vi "Get Waveform.vi"(0 "VISA resource name":refnum<visa-resource-name>, 1 "First Valid Point":i32, 2 "Last Valid Point":i32, 5 "Source (1: Channel 1)":u16(ring)=1 items=["Channel 1"=1, "Channel 2"=2, "Channel 3"=3, "Channel 4"=4], 7 "Command type (0: byte)":u16(ring) items=["Byte", "Word"], 9 "Number Of Data Points (10000)":i32=10000, 11 "error in (no error)":errorcluster, 12 "Timeout (10000 ms)":u32=10000, 13 "Array (0: DAT1)":u16(ring) items=["DAT1", "DAT2"]) -> (4 "VISA resource name out":refnum<visa-resource-name>, 6 "Waveform Graph":i16[](graph), 15 "error out":errorcluster)   [LabVIEW 2021, in "Siglent SDS 1000 2000 Series.lvlib"]
doc: "Read acquisition waveform from specified source and data block and command format."
uses:
  <instrlib>/Siglent SDS 1000 2000 Series/Siglent SDS 1000 2000 Series.lvlib
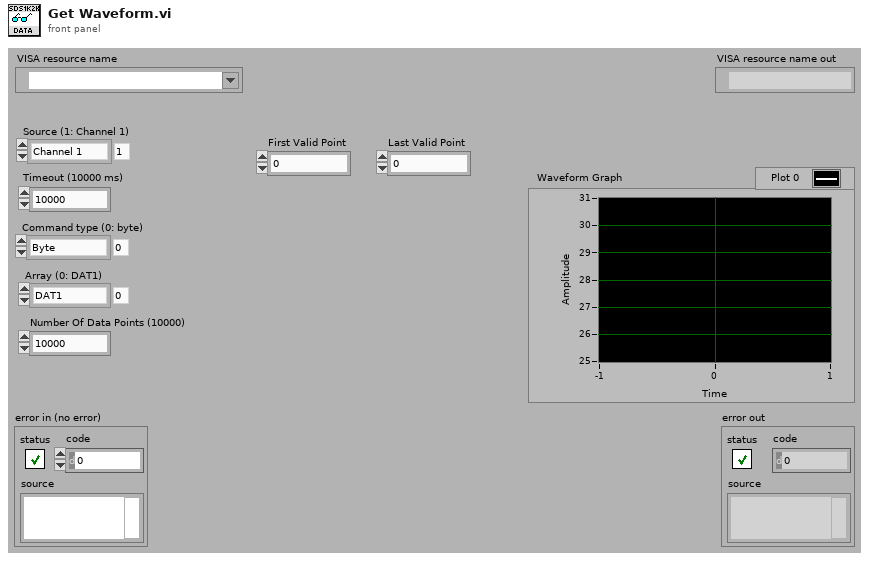
[diagram p1: front panel]
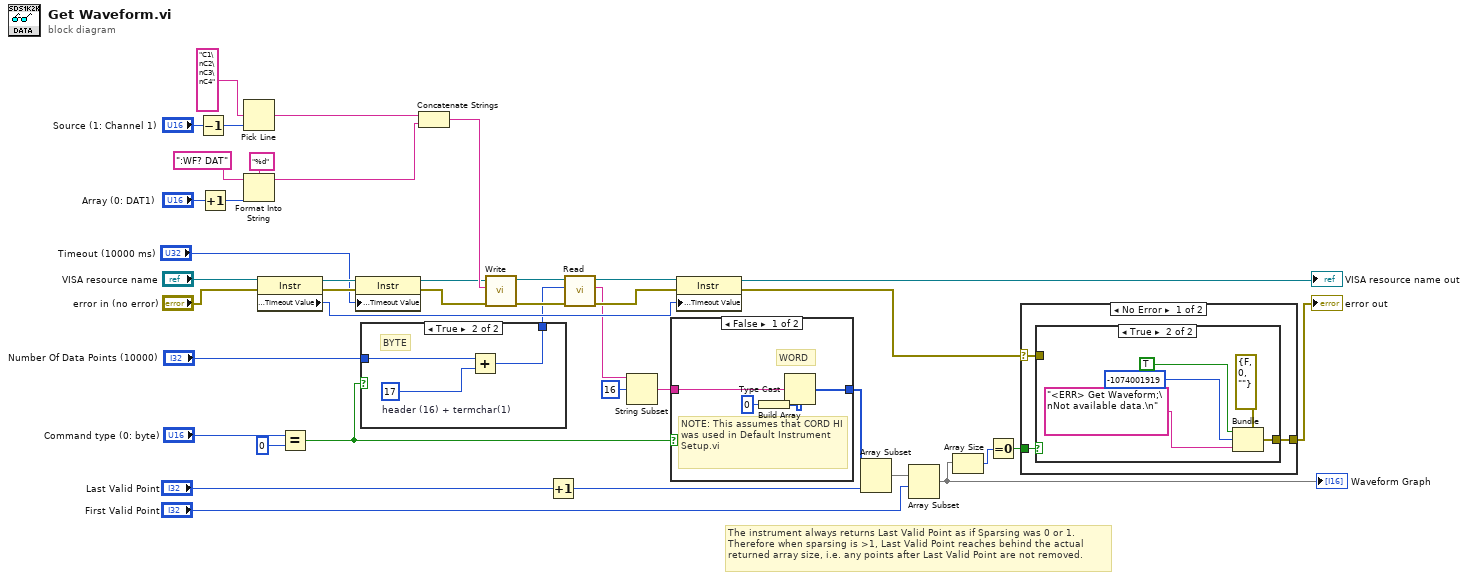
[diagram p0: block diagram]
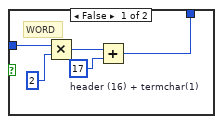
[diagram p4: hidden frame]
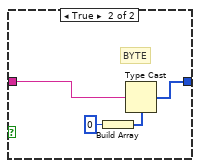
[diagram p5: hidden frame]
diagram:
  # "The instrument always returns Last Valid Point as if Sparsing was 0 or 1.\nTherefore when sparsing is >1, Last Valid Point reaches behind the actual\nreturned array size, i.e. any points after Last Valid Point are not removed."
  n1 = Decrement(x="Source (1: Channel 1)") -> (x-1=w1:u16)
  n2 = Increment(x="Array (0: DAT1)") -> (x+1=w20:u16)
  n3 = Pick Line(multi-line string="C1\nC2\nC3\nC4", line index=w1) -> (output string=w3:string)  [unwired: 1 in]
  n4 = Format Into String(format string="%d", initial string=":WF? DAT" ("write buffer"), w20) -> (resulting string=w33:string)  [unwired: 1 in, 1 out]
  n5 = property on="Property Node" class="Instr"(reference="VISA resource name", error in="error in (no error)") -> (reference out=w30:refnum<visa-resource-name>, error out=w29:errorcluster, "General Settings:Timeout Value"=w23:u32)
  n6 = Equal?(x="Command type (0: byte)", y=u16 0) -> (x = y?=w18:bool)
  n7 = property on="Property Node" class="Instr"(reference=w30, error in=w29, "General Settings:Timeout Value"="Timeout (10000 ms)") -> (reference out=w28:refnum<visa-resource-name>, error out=w27:errorcluster)
  n8 = case shown="True" w18 {
    tunnel: [w43 w48] -> w19
    tunnel: "Number Of Data Points (10000)" -> [w42 w47]
    frame False {
      w44 = 17  # header (16) + termchar(1)
      # "WORD"
      n9 = Multiply(x=w42, y=2) -> (x*y=w45:i32)
      n10 = Add(x=w45, y=w44) -> (x+y=w43:i32)
    }
    frame True {
      w49 = 17  # header (16) + termchar(1)
      # "BYTE"
      n11 = Add(x=w47, y=w49) -> (x+y=w48:i32)
    }
  }
  n12 = Concatenate Strings(w3, w33) -> (w41:string)
  n13 = call <instrlib>:"Write.vi"("error in (no error)"=w27, "Write Buffer"=w41, "VISA resource name"=w28) -> ("error out"=w39:errorcluster, "VISA resource name out"=w40:refnum<visa-resource-name>)  [unwired: 6 in, 1 out]
  n14 = Increment(x="Last Valid Point") -> (x+1=w4:i32)
  n15 = call <instrlib>:"Read.vi"("error in (no error)"=w39, "Byte Count"=w19, "VISA resource name"=w40) -> ("error out"=w25:errorcluster, "Read Buffer"=w6:string, "VISA resource name out"=w26:refnum<visa-resource-name>)  [unwired: 5 in, 1 out]
  n16 = String Subset(string=w6, offset (0)=16) -> (substring=w5:string)  [unwired: 1 in]
  n17 = case shown="False" w18 {
    tunnel: [w51 w55] -> w13
    tunnel: w5 -> [w50 w54]
    frame False {
      # "NOTE: This assumes that CORD HI was used in Default Instrument Setup.vi"
      # "WORD"
      n18 = Build Array(i16 0) -> (w52:i16[])
      n19 = Type Cast(type=w52, x=w50) -> (*(type *) &x=w51:i16[])
    }
    frame True {
      # "BYTE"
      n20 = Build Array(i8 0) -> (w56:i8[])
      n21 = Type Cast(type=w56, x=w54) -> (*(type *) &x=w55:i8[])
    }
  }
  n22 = property on="Property Node" class="Instr"(reference=w26, error in=w25, "General Settings:Timeout Value"=w23) -> (reference out=→"VISA resource name out":refnum<visa-resource-name>, error out=w9:errorcluster)
  n23 = Array Subset(array=w13, length=w4) -> (w16:i16[])  [unwired: 1 in]
  n24 = Array Subset(array=w16, index="First Valid Point") -> (w11:i16[])  [unwired: 1 in]
  "Waveform Graph" <- w11
  n25 = Array Size(array=w11) -> (size(s)=w10:i32)
  n26 = Equal To 0?(x=w10) -> (x = 0?=w8:bool)
  n27 = case shown="No Error" w9 {
    selector: w9 -> [w58 w67]
    tunnel: [w60 w67] -> w12
    tunnel: w8 -> [w59 _]
    frame No Error {
      n28 = case shown="True" w59 {
        tunnel: [w61 w62] -> w60
        tunnel: w58 -> [w61 _]
        frame False {
        }
        frame True {
          n29 = Bundle(cluster=errorcluster {"status"=FALSE, "code"=0, "source"=""} ("error out"), "status"=TRUE, "code"=-1074001919 ("Code"), "source"="<ERR> Get Waveform;\nNot available data.\n" ("Source")) -> (w62:errorcluster)
        }
      }
    }
    frame Error {
    }
  }
  "error out" <- w12
